vi "Class DVR API Generator.vi"() -> ()   [LabVIEW 2016]
doc: "A wrapper engine for generating DVR APIs for class methods."
uses:
  <vilib>/Utility/error.llb/DialogType.ctl
  SLL Queued State Machine/Queue Driver/Create Queue.vi
  SLL Queued State Machine/Queue Driver/Enqueue an Item to Queue.vi
  SLL Queued State Machine/Queue Driver/Dequeue Queue.vi
  SLL Queued State Machine/Queue Driver/Enqueue N Items.vi
  SLL Queued State Machine/Queue Driver/Flush Queue.vi
  SLL Queued State Machine/Queue Driver/Release Queue.vi
  SLL Queued State Machine/SLL QSM.lvlib
  SLL Scripting/SLL Scripting.lvlib
panel:
  out "Status":string
  in  "Run":bool
  in  "Method Folder Name":string="Methods"
  in  "DVR API Folder Name":string="APIs"
  in  "Class Path":path
  in  "DVR API Suffix":string=" API"
  # "Class DVR API Generator"
  # "Generates DVR based APIs for class methods. \n\nSpecify the \n1. Class path, \n2. Methods folder where the class methods are present,\n3. DVR API folder where the DVR APIs needs to be created,\n4. Suffix for the DVR APIs to be generated"
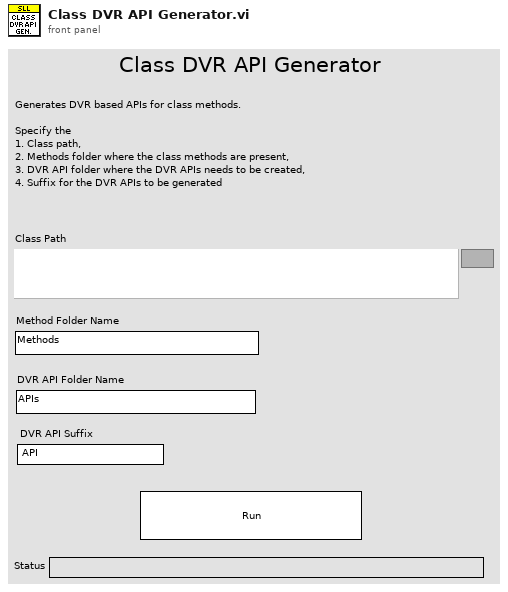
[diagram p1: front panel]
types:
  T1 = typedef "DialogType.ctl" = u16
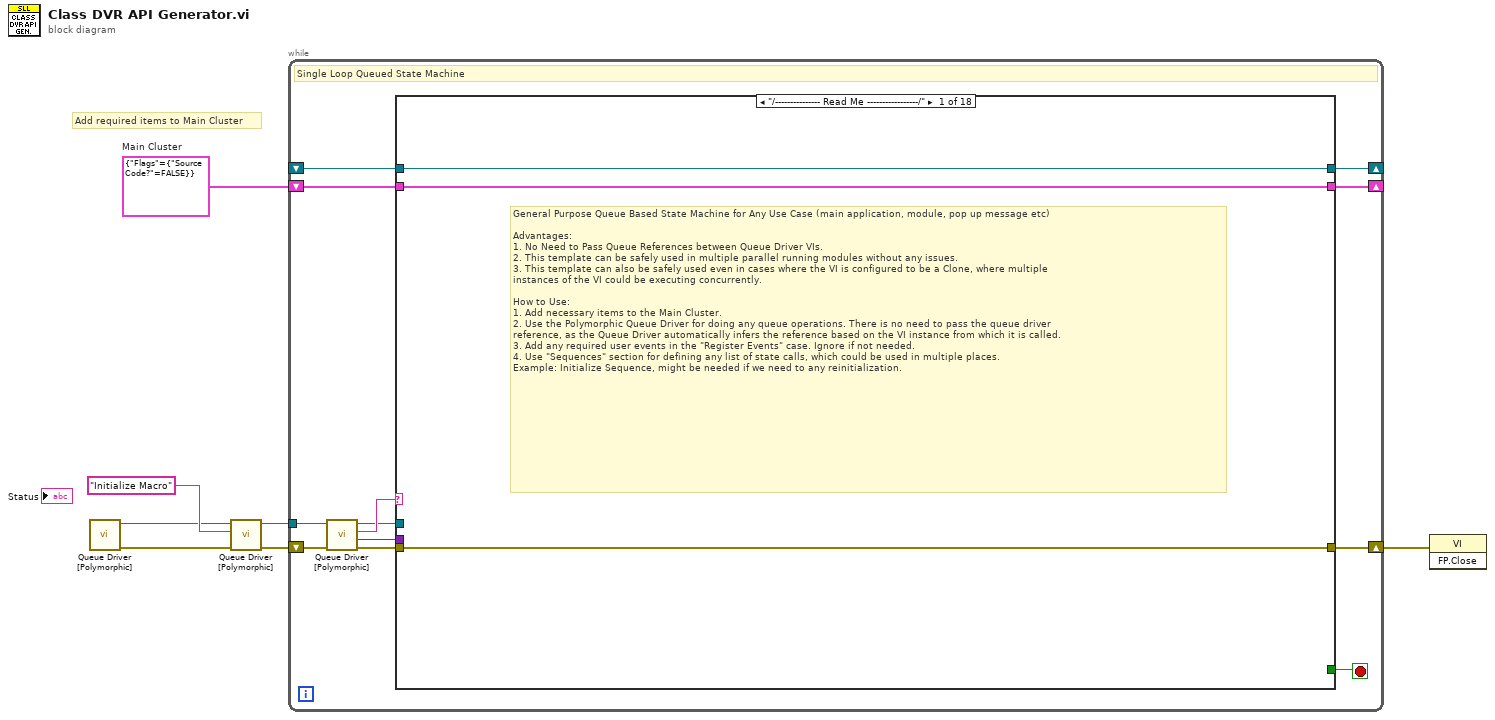
[diagram p0: block diagram]
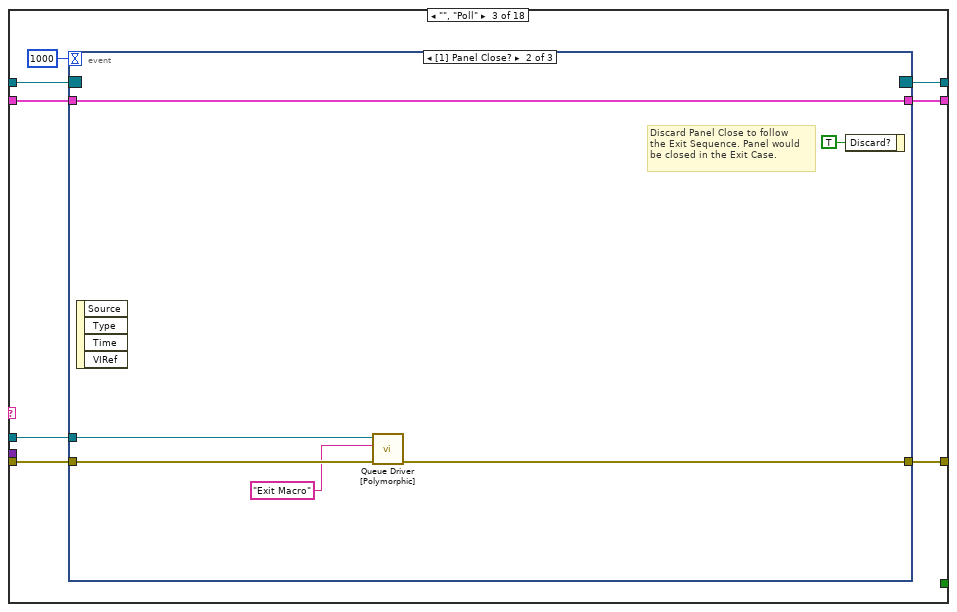
[diagram p3: hidden frame]
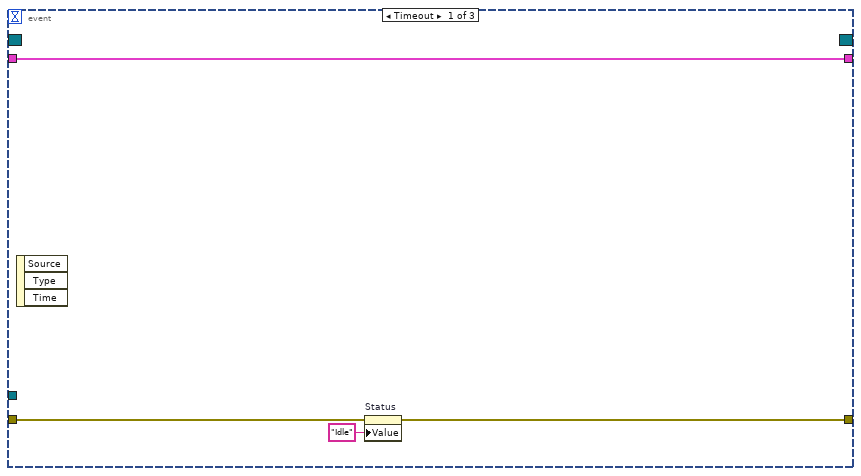
[diagram p4: hidden frame]
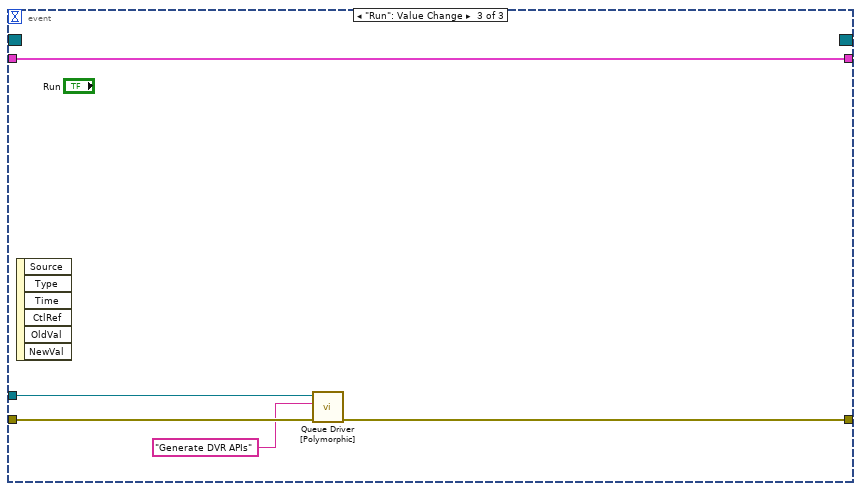
[diagram p5: hidden frame]
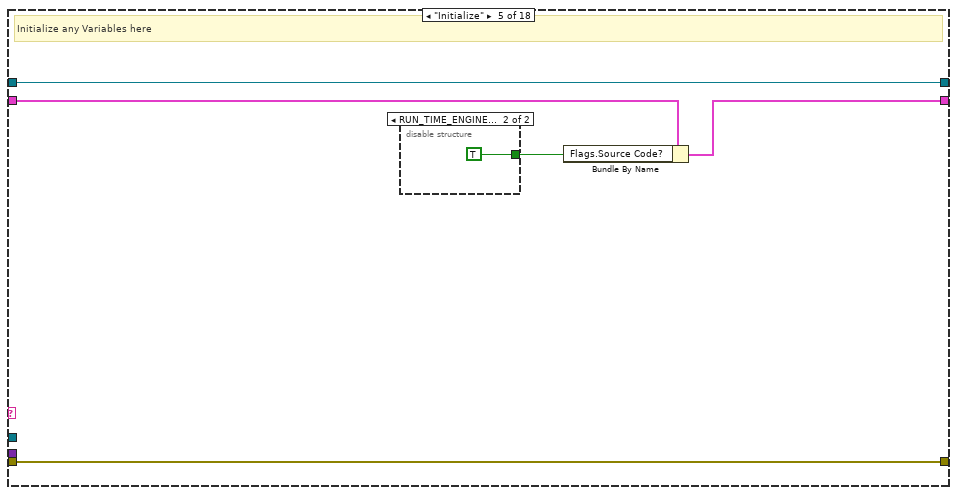
[diagram p7: hidden frame]
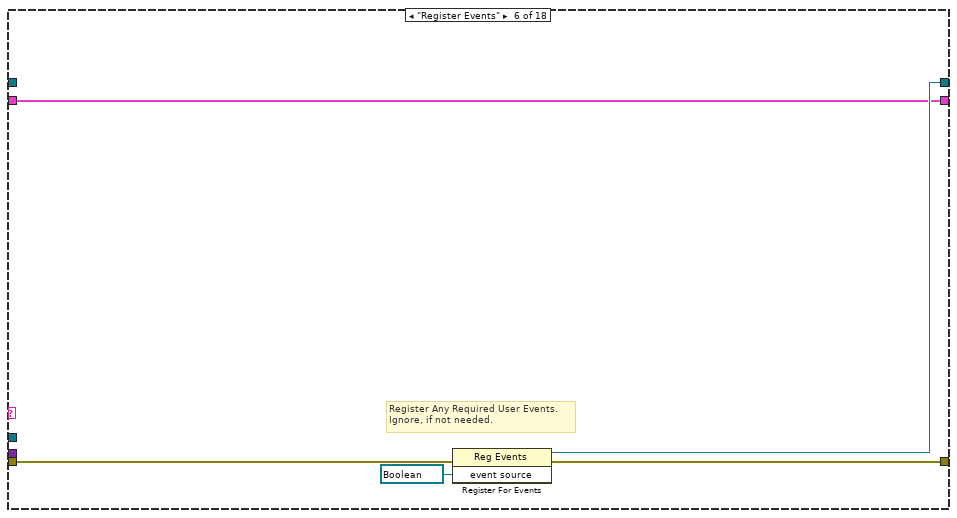
[diagram p9: hidden frame]
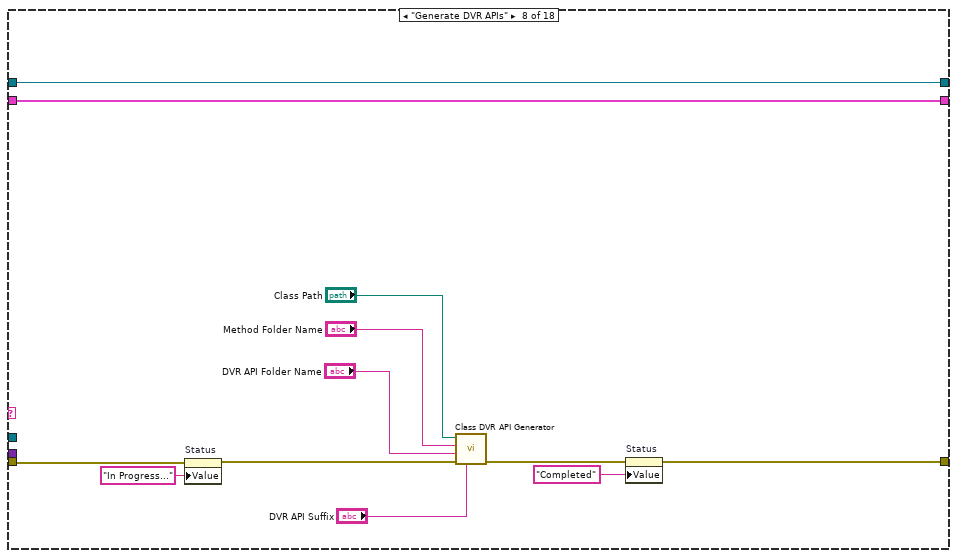
[diagram p11: hidden frame]
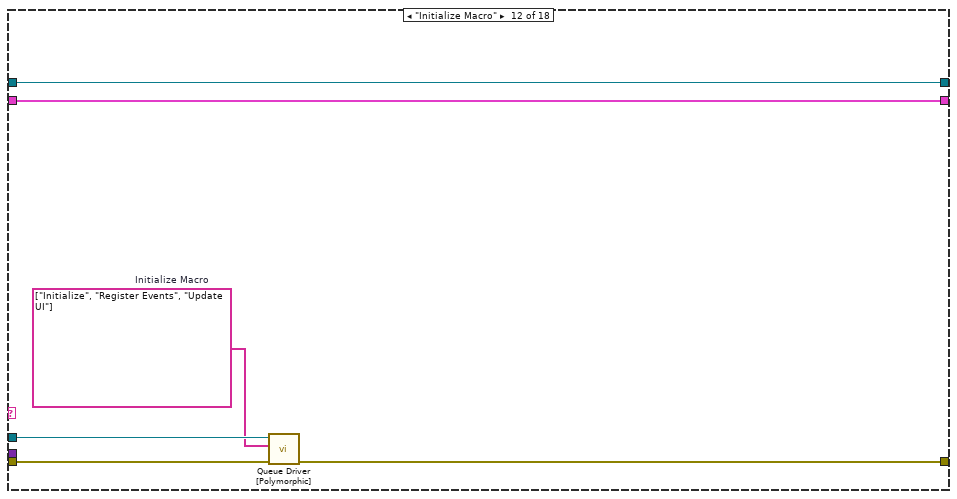
[diagram p15: hidden frame]
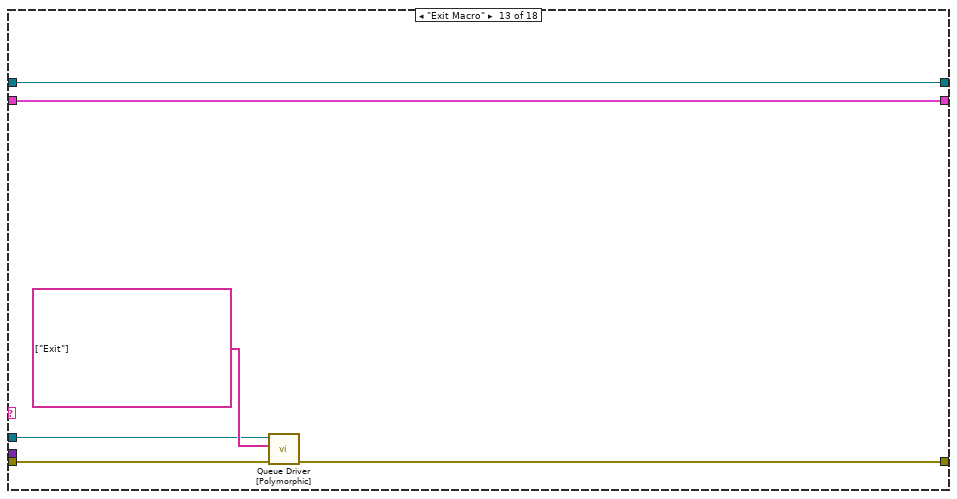
[diagram p16: hidden frame]
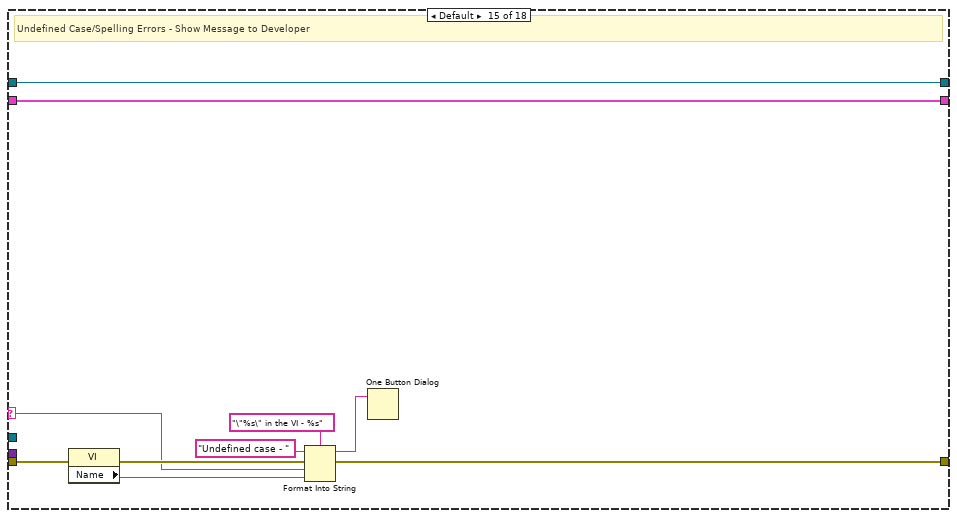
[diagram p18: hidden frame]
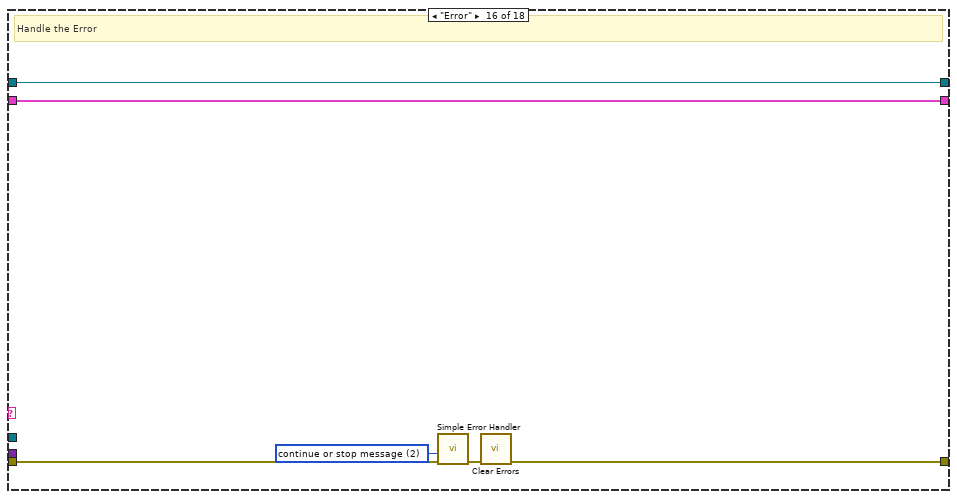
[diagram p19: hidden frame]
diagram:
  w5 = cluster{"Flags":cluster{"Source Code?":bool}} {"Flags"={"Source Code?"=FALSE}}  # Main Cluster
  # "Add required items to Main Cluster"
  n1 = call-poly "Queue Driver [Polymorphic].vi"() -> ("Error Out"=w7:errorcluster, "Queue Ref"=w3:refnum<queue>)  [unwired: 10 in]
  n2 = call-poly "Queue Driver [Polymorphic].vi"("Error In"=w7, "Item to Add"="Initialize Macro", "Queue Ref In"=w3) -> ("Error Out"=w6:errorcluster, "Queue Ref Out"=w2:refnum<queue>)  [unwired: 7 in]
  n3 = while "SLL Queued State Machine" {
    shift-right: [w17] -> w1
    shift-left: w6 -> [w19]
    shift-right: [w15] -> _
    shift-left: _ -> [w14]
    shift-right: [w13] -> _
    shift-left: w5 -> [w12]
    tunnel: w2 -> [w10]
    stop <- w16 stop-if-true
    # "Single Loop Queued State Machine"
    n4 = call-poly "Queue Driver [Polymorphic].vi"("Error In"=w19, "Queue Ref In"=w10) -> ("Error Out"=w18:errorcluster, "Data"=w8:variant, "Dequeue"=w11:string, "Queue Ref Out"=w9:refnum<queue>)  [unwired: 6 in]
    n5 = case "QSM Case Structure" shown="\"/--------------- Read Me -----------------/\"" w11 {
      selector: w11 -> [_ _ _ _ _ _ _ _ _ _ _ _ _ _ w102 _ _ _]
      tunnel: w18 -> [w22 w25 w31 w51 w56 w62 w65 w70 w80 w83 w86 w90 w96 w101 w105 w117 w120 w133]
      tunnel: [w22 w25 w32 w51 w56 w61 w65 w67 w80 w83 w86 w89 w95 w101 w108 w115 w120 w129] -> w17
      tunnel: [_ _ _ _ _ _ _ _ _ _ _ _ _ _ _ _ _ TRUE] -> w16
      tunnel: [w21 w24 w30 w50 w55 w60 w64 w77 w79 w82 w85 w92 w98 w100 w111 w114 w119 w132] -> w15
      tunnel: w14 -> [w21 w24 w29 w50 w55 _ w64 w77 w79 w82 w85 w92 w98 w100 w111 w114 w119 w132]
      tunnel: [w20 w23 w27 w49 w52 w59 w63 w76 w78 w81 w84 w91 w97 w99 w110 w113 w118 w131] -> w13
      tunnel: w12 -> [w20 w23 w28 w49 w53 w59 w63 w76 w78 w81 w84 w91 w97 w99 w110 w113 w118 w131]
      tunnel: w9 -> [_ _ w26 _ _ _ _ _ _ _ _ w88 w93 _ _ _ _ w122]
      tunnel: w8 -> [_ _ _ _ _ _ _ _ _ _ _ _ _ _ _ _ _ _]
      frame "/--------------- Read Me -----------------/" {
        # "General Purpose Queue Based State Machine for Any Use Case (main application, module, pop up message etc)\n\nAdvantages:\n1. No Need to Pass Queue References between Queue Driver VIs.\n2. This template can be safely used in multiple parallel running modules without any issues.\n3. This template can also be safely used even in cases where the VI is configured to be a Clone, where multiple \ninstances of the VI could be executing concurrently.\n\nHow to Use:\n1. Add necessary items to the Main Cluster.\n2. Use the Polymorphic Queue Driver for doing any queue operations. There is no need to pass the queue driver\nreference, as the Queue Driver automatically infers the reference based on the VI instance from which it is called.\n3. Add any required user events in the \"Register Events\" case. Ignore if not needed.\n4. Use \"Sequences\" section for defining any list of state calls, which could be used in multiple places. \nExample: Initialize Sequence, might be needed if we need to any reinitialization."
      }
      frame "/------------------ Poll -------------------/" {
      }
      frame "", "Poll" {
        n6 = event shown="[1] Panel Close?" {
          selector: w29 -> [_ _ _]
          dyn-events: [_ _ _] -> w30
          timeout: 1000 -> [_ _ _]
          tunnel: [w34 w42 w47] -> w32
          tunnel: w31 -> [w35 w43 w48]
          tunnel: w28 -> [w37 w41 w46]
          tunnel: [w37 w41 w46] -> w27
          tunnel: w26 -> [_ w38 w44]
          event Timeout {
            n7 = event-data() -> ()  [unwired: 1 in, 3 out]
            n8 = property on="Status" class="Str"(error in=w35, "Value"="Idle" ("Status")) -> (error out=w34:errorcluster)  [unwired: 1 in, 1 out]
          }
          event Panel Close? {
            # "Discard Panel Close to follow\nthe Exit Sequence. Panel would\nbe closed in the Exit Case."
            n9 = event-data() -> ()  [unwired: 1 in, 4 out]
            n10 = call-poly "Queue Driver [Polymorphic].vi"("Error In"=w43, "Item to Add"="Exit Macro" ("Enqueue"), "Queue Ref In"=w38) -> ("Error Out"=w42:errorcluster)  [unwired: 7 in, 1 out]
            n11 = event-data("Discard?"=TRUE) -> ()  [unwired: 1 in, 1 out]
          }
          event "Run": Value Change {
            n12 = event-data() -> ()  [unwired: 1 in, 6 out]
            n13 = call-poly "Queue Driver [Polymorphic].vi"("Error In"=w48, "Item to Add"="Generate DVR APIs" ("Enqueue"), "Queue Ref In"=w44) -> ("Error Out"=w47:errorcluster)  [unwired: 7 in, 1 out]
          }
        }
      }
      frame "/--------------- Initialize -----------------/" {
      }
      frame "Initialize" {
        # "Initialize any Variables here"
        n14 = disable-structure shown="RUN_TIME_ENGINE==False" {
          disable-tunnel: [_ TRUE] -> w54
          frame condition #0 {
          }
          frame condition #1 (active) {
          }
        }
        n15 = Bundle By Name(cluster=w53, "Flags.Source Code?"=w54) -> (w52:cluster{"Flags":cluster{"Source Code?":bool}})
      }
      frame "Register Events" {
        # "Register Any Required User Events. \nIgnore, if not needed."
        n16 = register-events(error in=w62, refnum<vi> refnum ("event source")) -> (reference out=w60:refnum<event-registration>, error out=w61:errorcluster)  [unwired: 1 in]
      }
      frame "/---------- Custom Case Splitter ----------/" {
      }
      frame "Generate DVR APIs" {
        n17 = property on="Status" class="Str"(error in=w70, "Value"="In Progress..." ("Status")) -> (error out=w71:errorcluster)  [unwired: 1 in, 1 out]
        n18 = call "Class DVR API Generator.vi"("DVR API Suffix"="DVR API Suffix", "error in (no error)"=w71, "DVR API Folder Name"="DVR API Folder Name", "Method Folder Name"="Method Folder Name", "Class Path"="Class Path") -> ("error out"=w68:errorcluster)  [unwired: 6 in]
        n19 = property on="Status" class="Str"(error in=w68, "Value"="Completed" ("Status")) -> (error out=w67:errorcluster)  [unwired: 1 in, 1 out]
      }
      frame "/-------------- User Interface --------------/" {
        # "Duplicate this case to create additional case splitters for readability"
      }
      frame "Update UI" {
        # "Update Front Panel Controls in this Case"
      }
      frame "/----------------- Macros -----------------/" {
      }
      frame "Initialize Macro" {
        w87 = string[] ["Initialize", "Register Events", "Update UI"]  # Initialize Macro
        n20 = call-poly "Queue Driver [Polymorphic].vi"("Error In"=w90, "Enqueue N"=w87, "Queue Ref In"=w88) -> ("Error Out"=w89:errorcluster)  [unwired: 7 in, 1 out]
      }
      frame "Exit Macro" {
        n21 = call-poly "Queue Driver [Polymorphic].vi"("Error In"=w96, "Enqueue N"=string[] ["Exit"], "Queue Ref In"=w93) -> ("Error Out"=w95:errorcluster)  [unwired: 7 in, 1 out]
      }
      frame "/-------------- Error Handler--------------/" {
      }
      frame Default {
        # "Undefined Case/Spelling Errors - Show Message to Developer"
        n22 = property class="VI"(error in=w105) -> (error out=w104:errorcluster, "Name"=w103:string)  [unwired: 1 in, 1 out]
        n23 = Format Into String(format string="\"%s\" in the VI - %s" ("message"), initial string="Undefined case - ", error in=w104, w102, w103) -> (resulting string=w106:string, error out=w108:errorcluster)
        n24 = One Button Dialog(message=w106) -> ()  [unwired: 1 in, 1 out]
      }
      frame "Error" {
        w112 = T1 2 items=["no dialog", "OK message", "continue or stop message", "OK message + warnings", "continue/stop + warnings"] ("type of dialog (OK msg:1)")
        # "Handle the Error"
        n25 = call <vilib>:"Simple Error Handler.vi"("type of dialog (OK msg:1)"=w112, "error in (no error)"=w117) -> ("error out"=w116:errorcluster)  [unwired: 3 in, 4 out]
        n26 = call <vilib>:"Clear Errors.vi"("error in (no error)"=w116) -> ("error out"=w115:errorcluster)  [unwired: 5 in, 1 out]
      }
      frame "/------------------- Exit --------------------/" {
      }
      frame "Exit" {
        n27 = call-poly "Queue Driver [Polymorphic].vi"("Error In"=w133, "Queue Ref In"=w122) -> ("Error Out"=w134:errorcluster, "Queue Ref Out"=w121:refnum<queue>)  [unwired: 7 in, 1 out]
        n28 = Unbundle By Name(w131) -> ("Flags.Source Code?"=w124:bool)
        n29 = call-poly "Queue Driver [Polymorphic].vi"("Error In"=w134, "Queue Ref In"=w121) -> ("Error Out"=w130:errorcluster)  [unwired: 9 in]
        n30 = Call Chain() -> (call chain=w128:string[])
        n31 = Array Size(array=w128) -> (size(s)=w127:i32)
        n32 = Equal?(x=w127, y=1) -> (x = y?=w125:bool)
        n33 = And(x=w124, y=w125) -> (x .and. y?=w123:bool)
        n34 = case "Skip Panel Close when in Source\nCode and is the top most caller" shown="True" w123 {
          tunnel: w130 -> [w137 w139]
          tunnel: [w138 w139] -> w129
          frame False {
            # "Close Panel"
            n35 = invoke class="VI" method="FP.Close"() -> (error out=w136:errorcluster)  [unwired: 3 in, 2 out]
            n36 = Merge Errors(w137, w136) -> (w138:errorcluster)
          }
          frame True {
            # "Do Not Close Panel"
          }
        }
      }
    }
  }
  n37 = invoke class="VI" method="FP.Close"(error in=w1) -> ()  [unwired: 2 in, 3 out]
